vi "get error.vi"(8 "error in":errorcluster, 11 "result in":refnum<class "result.lvclass">) -> (0 "error out":errorcluster, 2 "error":errorcluster, 3 "result out":refnum<class "result.lvclass">)   [LabVIEW 2013, in "result.lvclass"]
uses:
  result.lvclass
  result.lvclass/result.ctl
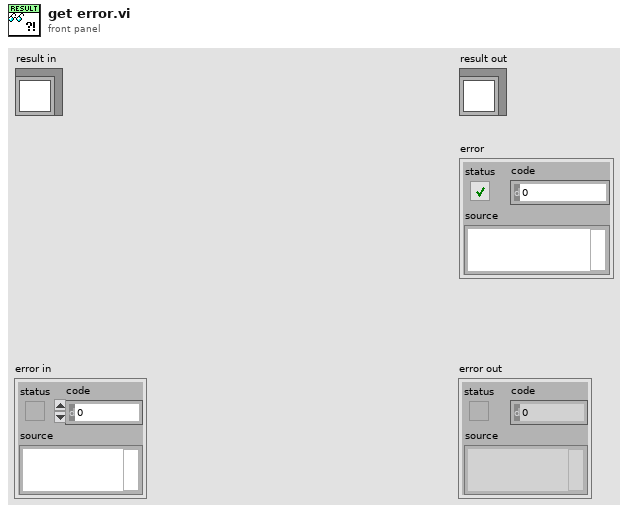
[diagram p1: front panel]
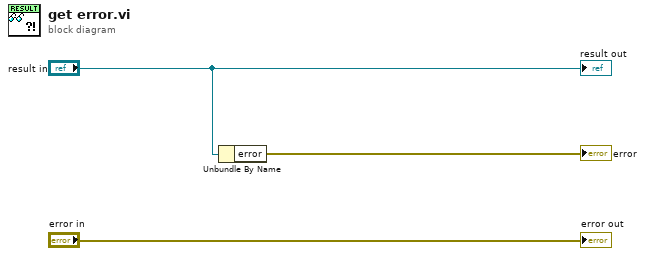
[diagram p0: block diagram]
diagram:
  n1 = Unbundle By Name("result in") -> ("error"=→"error":errorcluster)
  "error out" <- "error in"
  "result out" <- "result in"
